vi "Syringe Stepper Interlock Configuration.vi"(8 "error in (no error)":errorcluster, 11 "cRIO-CO2 in":refnum<class "cRIO-CO2.lvclass">) -> (0 "error out":errorcluster, 2 "Interlock Chain":refnum<class "Interlock Chain.lvclass">, 3 "cRIO-CO2 out":refnum<class "cRIO-CO2.lvclass">)   [LabVIEW 2015, in "cRIO-Carbondioxide.lvlib" / "cRIO-CO2.lvlib" / "cRIO-CO2.lvclass"]
uses:
  cRIO-CO2.lvclass
  Interlocks/Interlock Chain/Interlock Chain.lvclass
  Interlocks/Interlock/Interlock.lvclass
  Interlocks/Interlock Bool/Interlock Bool.lvclass
  Interlocks/Interlock Bool/Interlock Bool.lvclass/Interlock Bool.ctl
  Interlocks/Interlock Chain/Interlock Chain.lvclass/Interlock Chain.ctl
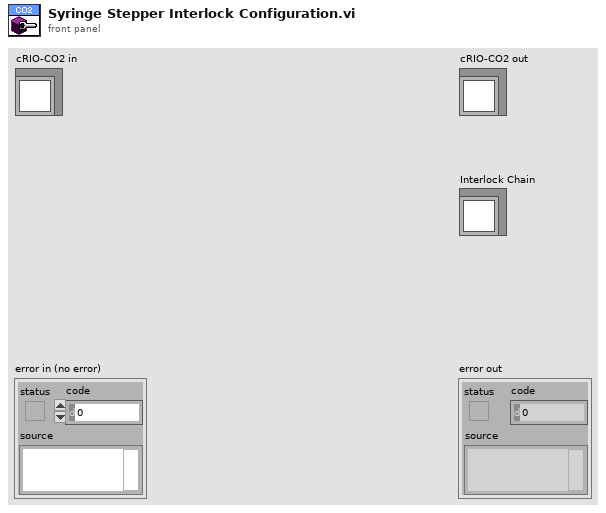
[diagram p1: front panel]
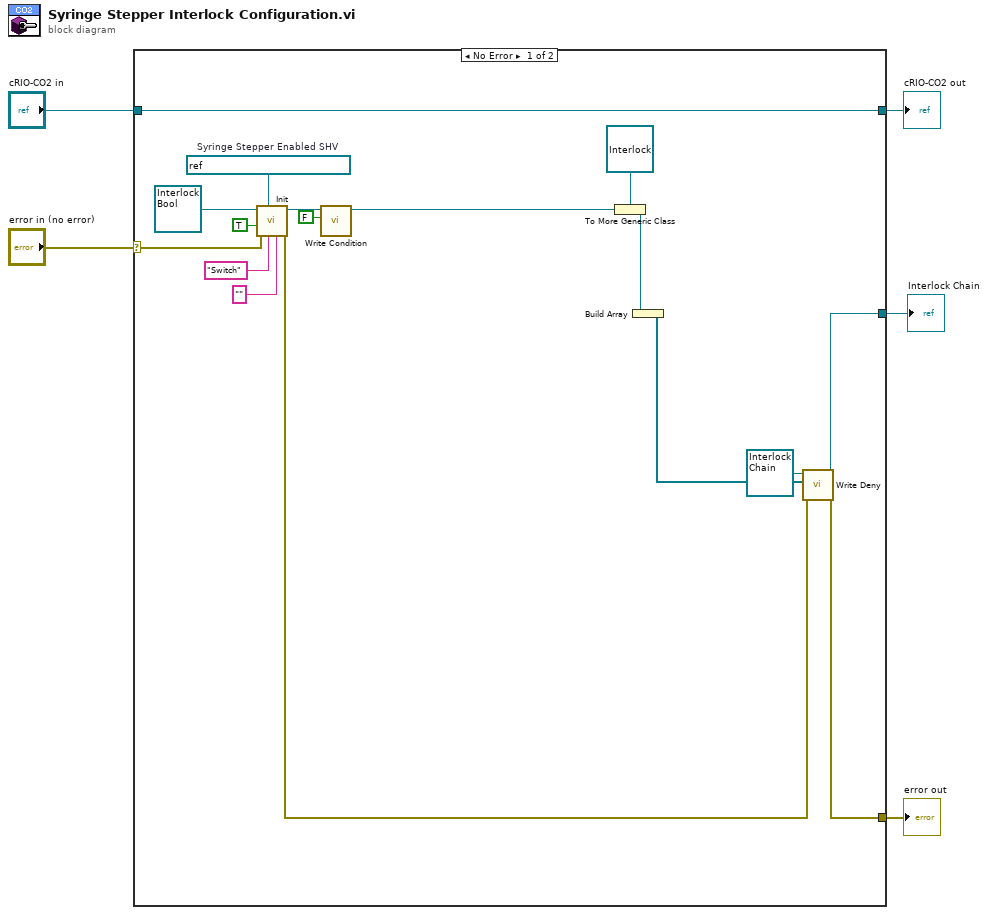
[diagram p0: block diagram]
diagram:
  n1 = case shown="No Error" "error in (no error)" {
    selector: "error in (no error)" -> [w17 w24]
    tunnel: [w9 w24] -> w4
    tunnel: [w22 w23] -> w2
    tunnel: "cRIO-CO2 in" -> [w22 w23]
    tunnel: [w7 _] -> w1
    frame No Error {
      w19 = refnum<k21> "ni.var.psp://10.2.0.20/AMS Gas SHV/Stepper/Enabled"  # Syringe Stepper Enabled SHV
      n2 = call-dynamic "Init.vi"("Interlock message (\" -> Interlock!\")"="" ("Interlock message (\" -> Interlock!\")"), "Name (SHV Name if empty)"="Switch", "SHV"=w19, "error in (no error)"=w17, "Stop Self on IL? (T)"=TRUE, "Interlock in"=refnum<class "Interlock Bool.lvclass"> refnum ("Interlock Bool.lvclass")) -> ("error out"=w10:errorcluster, "Interlock out"=w20:refnum<class "Interlock Bool.lvclass">)  [unwired: 4 in]
      n3 = call "Write Condition.vi"("Interlock Condition"=FALSE, "Interlock Bool in"=w20) -> ("Interlock Bool out"=w15:refnum<class "Interlock Bool.lvclass">)  [unwired: 8 in, 1 out]
      n4 = To More Generic Class(target class=refnum<class "Interlock.lvclass"> refnum ("Interlock.lvclass"), reference=w15) -> (generic class reference=w13:refnum<class "Interlock.lvclass">)
      n5 = Build Array(w13) -> (w8:refnum<class "Interlock.lvclass">[])
      n6 = call "Write Deny.vi"("error in (no error)"=w10, "Deny"=w8, "Interlock Chain in"=refnum<class "Interlock Chain.lvclass"> refnum) -> ("error out"=w9:errorcluster, "Interlock Chain out"=w7:refnum<class "Interlock Chain.lvclass">)  [unwired: 7 in]
    }
    frame Error {
    }
  }
  "error out" <- w4
  "cRIO-CO2 out" <- w2
  "Interlock Chain" <- w1
